vi "1_1_Botones.vi"() -> ()   [LabVIEW 2020]
panel:
  in  "Switch Stop":bool
  out "Accion 1":bool
  out "Acción 3":bool
  out "Acción 2":bool
  in  "Latch Stop":bool
  in  "Latch Stop":bool
  out "Acción 6":dbl
  in  "Latch until Released":bool
  out "Acción 4":dbl
  in  "Latch when Pressed":bool
  in  "Latch when Released":bool
  out "Acción 5":dbl
  in  "Latch Stop":bool
  in  "Switch until Released":bool
  in  "Switch when Released":bool
  in  "Switch when Pressed":bool
  # "1. Tipos de datos\n\n1.1 Elabore un programa donde muestre un ejemplo de cada uno de los modos de acción mecánica\nde los botones (6 modos). Considere que deberá ser claro para comprender para el usuario."
  # "Latch"
  # "Switch"
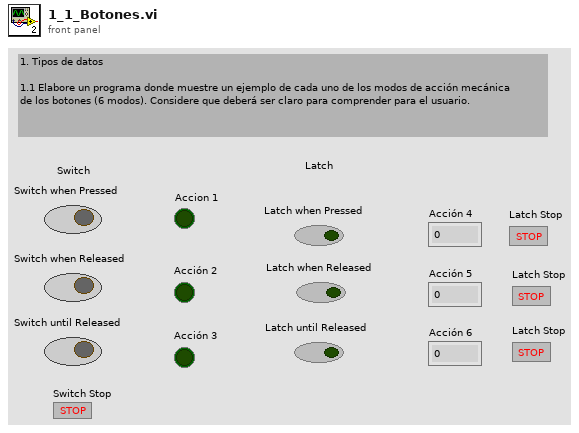
[diagram p1: front panel]
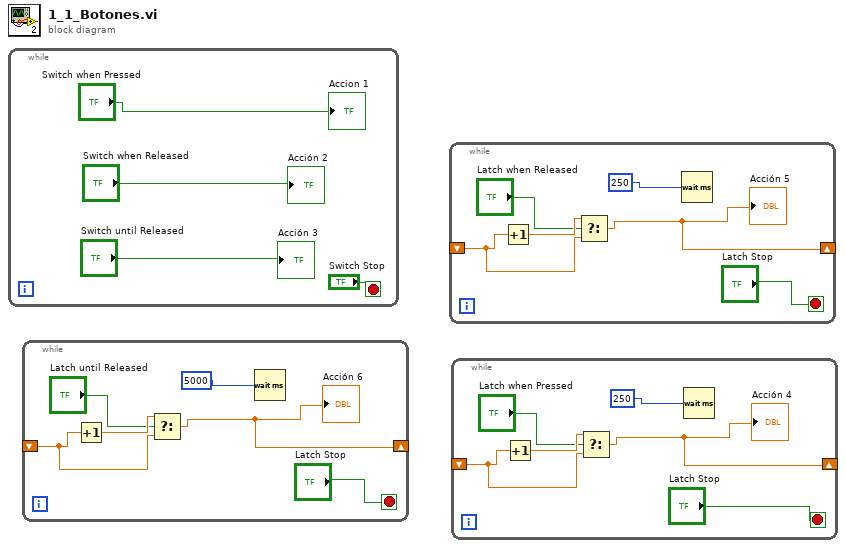
[diagram p0: block diagram]
diagram:
  n1 = while {
    stop <- "Switch Stop" stop-if-true
    "Acción 2" <- "Switch when Released"
    "Acción 3" <- "Switch until Released"
    "Accion 1" <- "Switch when Pressed"
  }
  n2 = while {
    shift-right: [w8] -> _
    shift-left: _ -> [w6]
    stop <- "Latch Stop" stop-if-true
    n3 = Increment(x=w6) -> (x+1=w7:dbl)
    n4 = Select(t=w7, s="Latch until Released", f=w6) -> (s? t:f=w8:dbl)
    "Acción 6" <- w8
    n5 = Wait (ms)(milliseconds to wait=5000) -> ()  [unwired: 1 out]
  }
  n6 = while {
    shift-right: [w14] -> _
    shift-left: _ -> [w12]
    stop <- "Latch Stop" stop-if-true
    n7 = Increment(x=w12) -> (x+1=w13:dbl)
    n8 = Select(t=w13, s="Latch when Released", f=w12) -> (s? t:f=w14:dbl)
    "Acción 5" <- w14
    n9 = Wait (ms)(milliseconds to wait=250) -> ()  [unwired: 1 out]
  }
  n10 = while {
    shift-right: [w21] -> _
    shift-left: _ -> [w19]
    stop <- "Latch Stop" stop-if-true
    n11 = Increment(x=w19) -> (x+1=w20:dbl)
    n12 = Select(t=w20, s="Latch when Pressed", f=w19) -> (s? t:f=w21:dbl)
    "Acción 4" <- w21
    n13 = Wait (ms)(milliseconds to wait=250) -> ()  [unwired: 1 out]
  }
